vi "Read from Execution Units.vi"(8 "error in (no error)":errorcluster, 11 "RTStateVariables in":T1 {"Execution Unit Runtime Information"."Outgoing Data References"."Data Reference" format="%.0x"; "Execution Unit Runtime Information"."Incoming Data References" format="%.0x"}) -> (0 "error out":errorcluster, 3 "RTStateVariables out":T1 {"Execution Unit Runtime Information"."Outgoing Data References"."Data Reference" format="%.0x"; "Execution Unit Runtime Information"."Incoming Data References" format="%.0x"})   [LabVIEW 2020, in "Communication Bus Template Engine.lvlib"]
uses:
  Communication Bus Template Engine.lvlib
  RTStateVariables.ctl
  <vilib>/NI/NIVS Inline Async API/_VS Inline Async API/VS Inline Async API/VS Inline Async API.lvclass
  Includes/Communication Bus Interfaces.lvlibp/Execution Unit/Execution Unit/Execution Unit.lvclass
  Execution Unit Runtime Information.ctl
  <vilib>/NI VeriStand/Custom Device API/Data Reference.ctl
  <vilib>/NI VeriStand/Custom Device API/Block Data Reference.ctl
  <vilib>/NI VeriStand/Custom Device API/Global Data Refs.vi
  <vilib>/NI VeriStand/Custom Device API/Custom Device API.lvlib
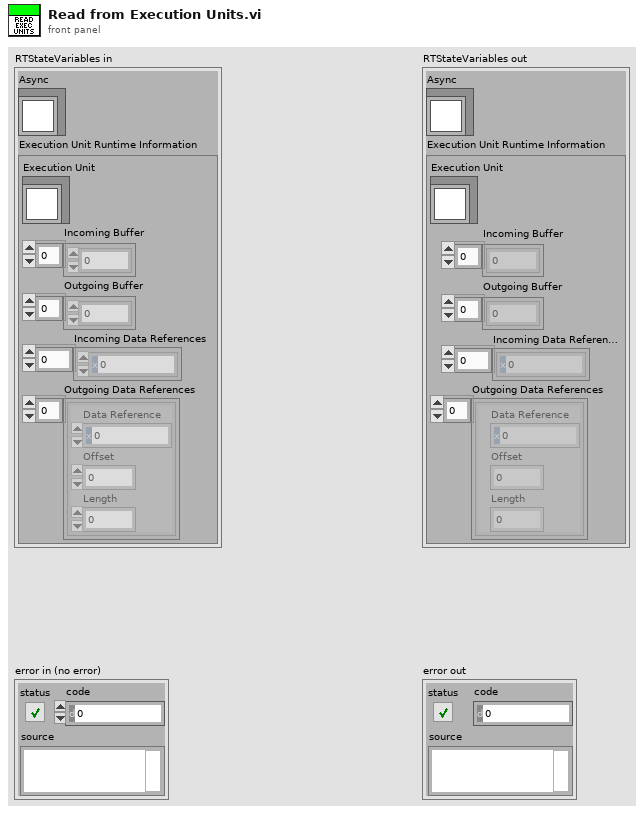
[diagram p1: front panel]
types:
  T1 = typedef "Communication Bus Template Engine.lvlib/RTStateVariables.ctl" = cluster{"Async":refnum<class "VS Inline Async API.lvclass">, "Execution Unit Runtime Information":T2}
  T2 = typedef "Communication Bus Template Engine.lvlib/Execution Unit Runtime Information.ctl" = cluster{"Execution Unit":refnum<class "Execution Unit.lvclass">, "Incoming Buffer":dbl[], "Outgoing Buffer":dbl[], "Incoming Data References":T3[], "Outgoing Data References":T4[]}
  T3 = typedef "Custom Device API.lvlib/Data Reference.ctl" = i32
  T4 = typedef "Custom Device API.lvlib/Block Data Reference.ctl" = cluster{"Data Reference":T3, "Offset":u64, "Length":u64}
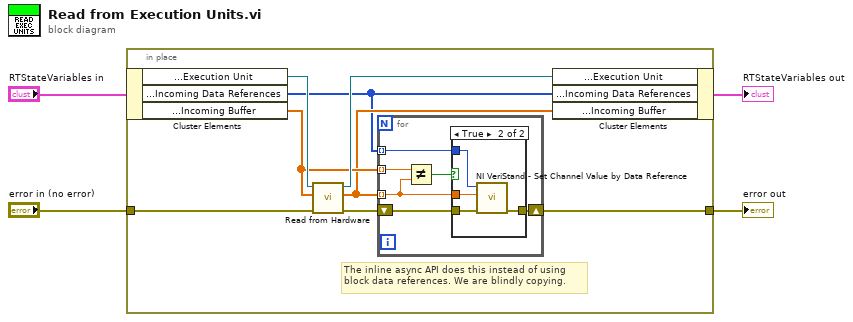
[diagram p0: block diagram]
diagram:
  n1 = in-place {
    in-place-border: "error in (no error)" -> [w10]
    in-place-border: [w6] -> w4
    # "The inline async API does this instead of using\nblock data references. We are blindly copying."
    n2 = in-place-cluster #1("RTStateVariables in") -> ("Execution Unit Runtime Information.Execution Unit"=w12:refnum<class "Execution Unit.lvclass">, "Execution Unit Runtime Information.Incoming Data References"=w5:T3[], "Execution Unit Runtime Information.Incoming Buffer"=w9:dbl[])
    n3 = call-dynamic "Read from Hardware.vi"("error in (no error)"=w10, "Values in"=w9, "Execution Unit in"=w12) -> ("error out"=w7:errorcluster, "Values out"=w8:dbl[], "Execution Unit out"=w11:refnum<class "Execution Unit.lvclass">)  [unwired: 6 in]
    n4 = for {
      tunnel: w9 -> [w15] mode=indexing
      tunnel: w8 -> [w14] mode=indexing
      shift-right: [w16] -> w6
      shift-left: w7 -> [w17]
      tunnel: w5 -> [w13] mode=indexing
      n5 = Not Equal?(x=w15, y=w14) -> (x != y?=w18:bool)
      n6 = case shown="True" w18 {
        tunnel: w17 -> [w19 w23]
        tunnel: [w19 w22] -> w16
        tunnel: w14 -> [_ w21]
        tunnel: w13 -> [_ w20]
        frame False {
        }
        frame True {
          n7 = call <vilib>:"NI VeriStand - Set Channel Value by Data Reference.vi"("error in (no error)"=w23, "Value"=w21, "Data Reference in"=w20) -> ("error out"=w22:errorcluster)  [unwired: 8 in]
        }
      }
    }
    n8 = in-place-cluster #1("Execution Unit Runtime Information.Execution Unit"=w11, "Execution Unit Runtime Information.Incoming Data References"=w5, "Execution Unit Runtime Information.Incoming Buffer"=w8) -> (→"RTStateVariables out":T1)
  }
  "error out" <- w4
